vi "2.2.-Lectura de Imagen - Operador Inverso.vi"() -> ()   [LabVIEW 2020]
panel:
  out "new picture":picture
  in  "Path":path
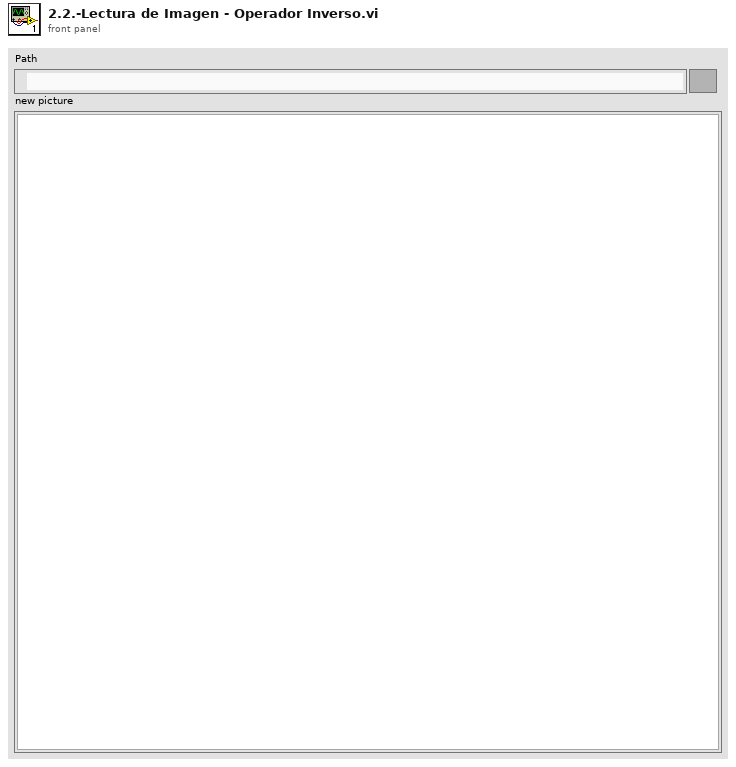
[diagram p1: front panel]
types:
  T1 = typedef "imagedata.ctl" = cluster{"image type":i32, "image depth":i32, "image":u8[], "mask":u8[], "colors":u32[], "Rectangle":cluster{"left":i16, "top":i16, "right":i16, "bottom":i16}}
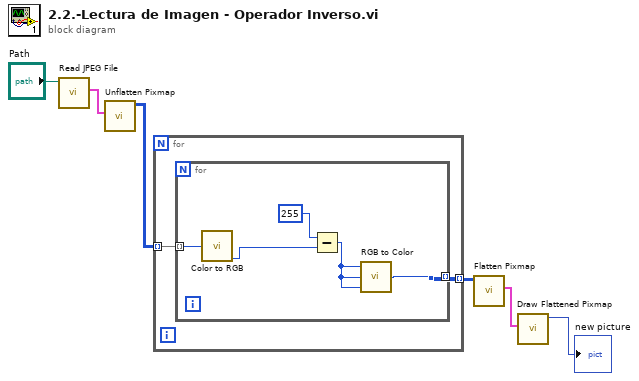
[diagram p0: block diagram]
diagram:
  n1 = call <vilib>:"Read JPEG File.vi"("path to JPEG file"="Path") -> ("image data"=w5:T1)  [unwired: 8 in, 2 out]
  n2 = call <vilib>:"Unflatten Pixmap.vi"("image data"=w5) -> ("24-bit pixmap"=w4:u32[][])  [unwired: 4 in, 6 out]
  n3 = for {
    tunnel: w4 -> [w8] mode=indexing
    tunnel: [w7] -> w3 mode=indexing
    n4 = for {
      tunnel: w8 -> [w13] mode=indexing
      tunnel: [w12] -> w7 mode=indexing
      n5 = call <vilib>:"Color to RGB.vi"("Color"=w13) -> ("B"=w10:u8)  [unwired: 3 out]
      n6 = Subtract(x=255, y=w10) -> (x-y=w9:i32)
      n7 = call <vilib>:"RGB to Color.vi"("B"=w9, "G"=w9, "R"=w9) -> ("Color"=w12:u32)
    }
  }
  n8 = call <vilib>:"Flatten Pixmap.vi"("24-bit pixmap"=w3) -> ("image data"=w2:T1)  [unwired: 10 in]
  n9 = call <vilib>:"Draw Flattened Pixmap.vi"("image data"=w2) -> ("new picture"=→"new picture":picture)  [unwired: 8 in]
